vi "main.vi"() -> ()   [LabVIEW 2015, in "example_01.lvlib"]
uses:
  example_01.lvlib
  _controls/recipes.ctl
  _controls/manual_actions.ctl
  lv-recipe-machine/public/_controls/configuration.ctl
  _controls/step_data.ctl
  lv-recipe-machine/public/_controls/mode.ctl
  lv-recipe-machine/lv-recipe-machine.lvlib
panel:
  out "error":errorcluster
  in  "refresh_rate_ms":i32=-1
  out "comparison":bool
  in  "wait_time_ms":i32=1000
  in  "stop":bool
  in  "manual_action":T1=enum."manual_test_random"
  in  "execute":bool
  in  "recipe":T2=enum."simple_random_and_wait"
  in  "resume":bool
  in  "abort":bool
  in  "pause":bool
  in  "start":bool
  in  "manual_mode":bool
  in  "automatic_mode":bool
  out "wait_elapsed_time":dbl format="%<%H:%M:%S%3u>t"
  out "recipe_elapsed_time":dbl format="%<%H:%M:%S>t"
  out "random_data":dbl
  out "action_step":string
  out "state":string
  out "mode":string
  in  "events":i32(listbox)=-1
  # "Manual Inputs"
  # "Automatic Inputs"
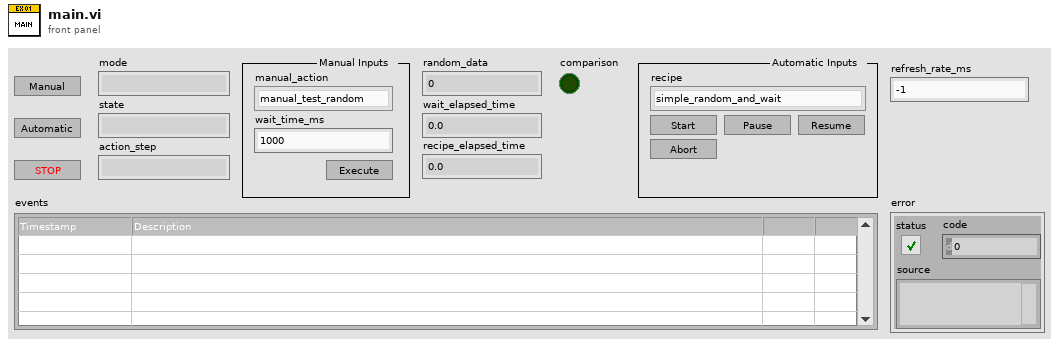
[diagram p1: front panel]
types:
  T1 = typedef "example_01.lvlib/manual_actions.ctl" = enum16{"<manual_action>", "manual_test_random", "manual_test_comparison", "manual_test_wait", "<null>"}
  T2 = typedef "example_01.lvlib/recipes.ctl" = enum16{"<recipes>", "simple_random_and_wait", "simple_random_and_test", "intermediate_fixed_continuous", "intermediate_test_with_continuous_fail", "<null>"}
  T3 = typedef "lv-recipe-machine.lvlib/configuration.ctl" = cluster{"max_processes":i32}
  T4 = typedef "lv-recipe-machine.lvlib/references.ctl" = cluster{"semaphore":T5, "input_queue":refnum<queue>, "output_queue":refnum<queue>, "data_dvr":refnum<data-value>, "stop_notifier":refnum<notifier>, "waitgroup_dvr":refnum<data-value>, "change_in_event":refnum<user-event>, "change_out_event":refnum<user-event>, "status_event":refnum<user-event>}
  T5 = typedef "Semaphore RefNum" = refnum<k1>
  T6 = typedef "example_01.lvlib/step_data.ctl" = cluster{"data":variant, "step":string}
  T7 = typedef "lv-recipe-machine.lvlib/mode.ctl" = enum16{"<mode>", "manual", "automatic", "<null>"}
  T8 = typedef "lv-recipe-machine.lvlib/status.ctl" = cluster{"mode":T7, "manual_state":T9, "automatic_state":T10, "step":string, "auto_elapsed_time":dbl}
  T9 = typedef "lv-recipe-machine.lvlib/manual_state.ctl" = enum16{"<manual_state>", "failed", "action", "running", "idle", "<null>"}
  T10 = typedef "lv-recipe-machine.lvlib/automatic_state.ctl" = enum16{"<automatic_state>", "failed", "idle", "running", "paused", "transition", "stopped", "<null>"}
  T11 = typedef "lv-recipe-machine.lvlib/recipe_step.ctl" = cluster{"step":string, "data":variant}
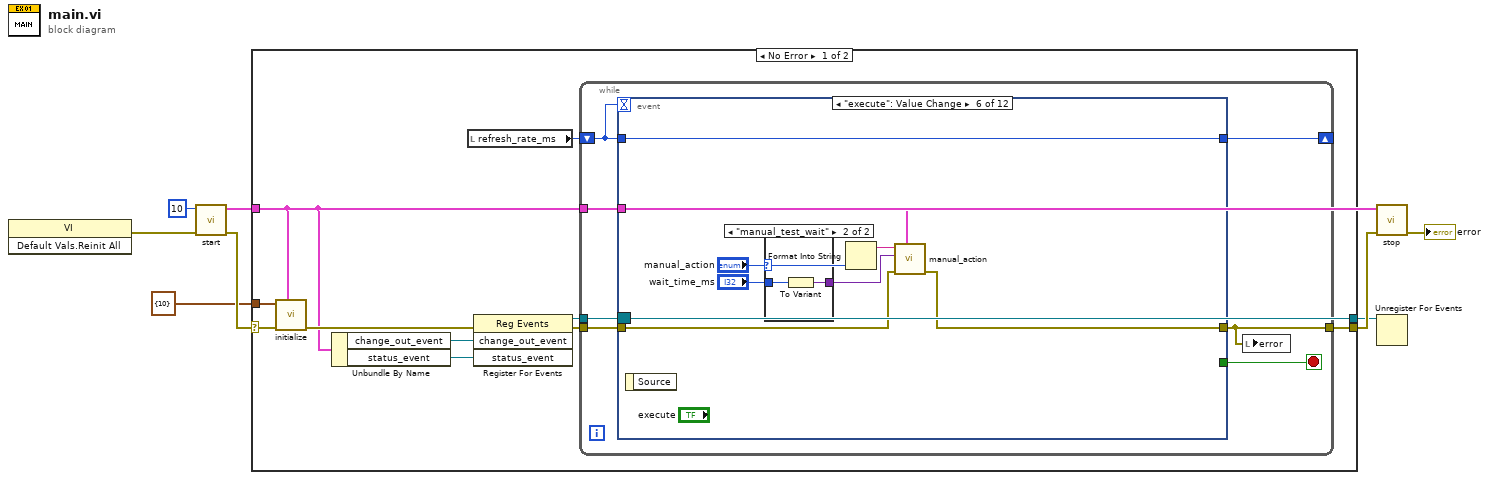
[diagram p0: block diagram]
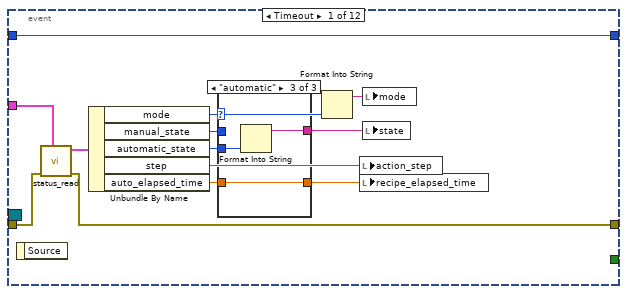
[diagram p2: hidden frame]
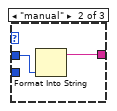
[diagram p4: hidden frame]
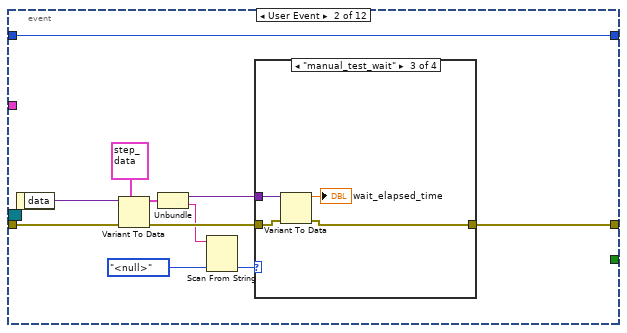
[diagram p5: hidden frame]
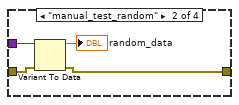
[diagram p7: hidden frame]
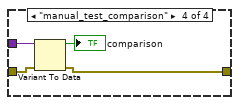
[diagram p8: hidden frame]
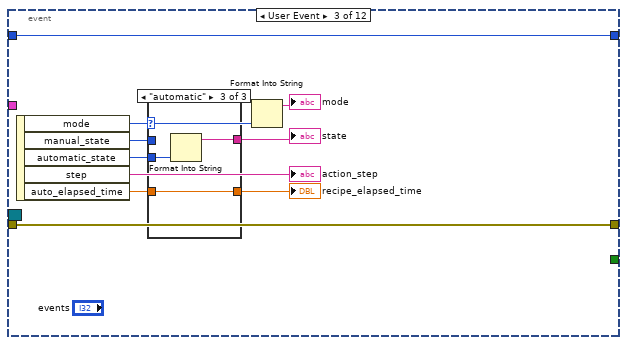
[diagram p9: hidden frame]
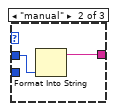
[diagram p11: hidden frame]
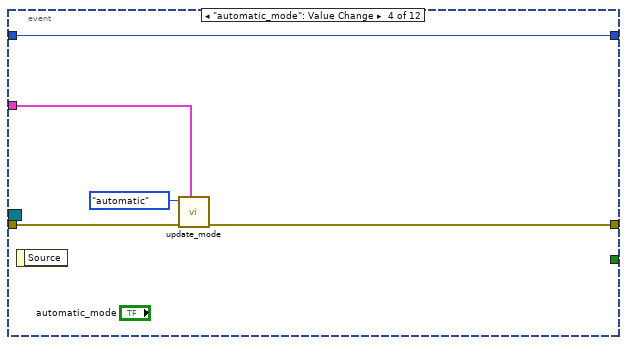
[diagram p12: hidden frame]
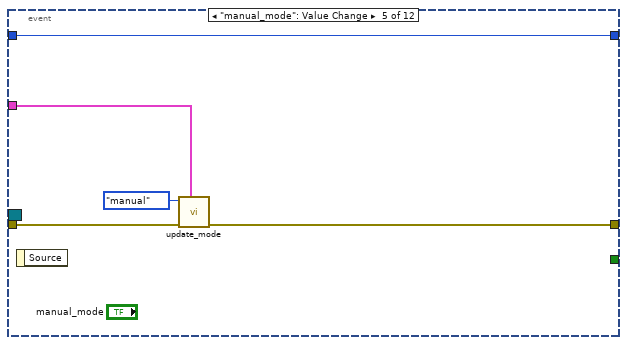
[diagram p13: hidden frame]
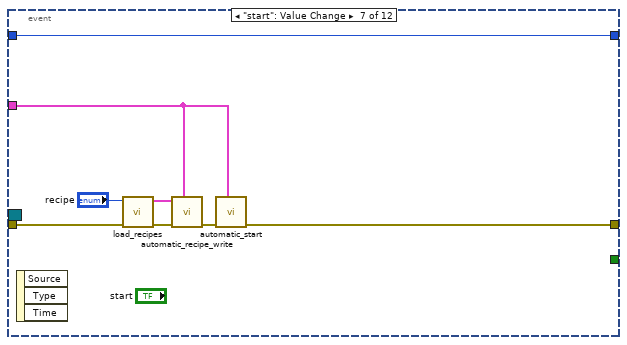
[diagram p15: hidden frame]
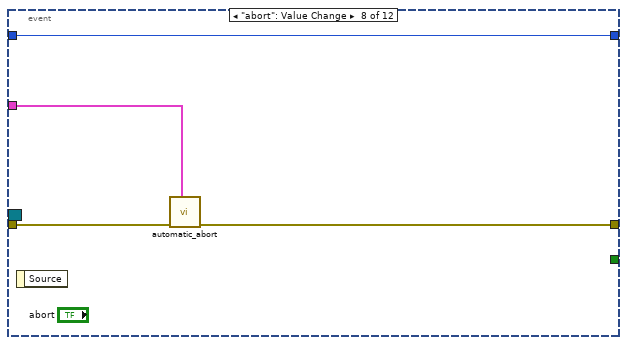
[diagram p16: hidden frame]
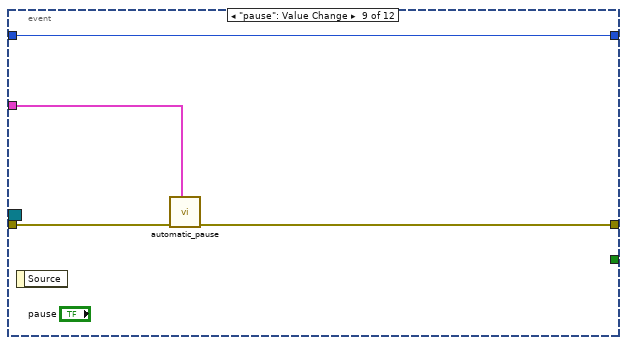
[diagram p17: hidden frame]
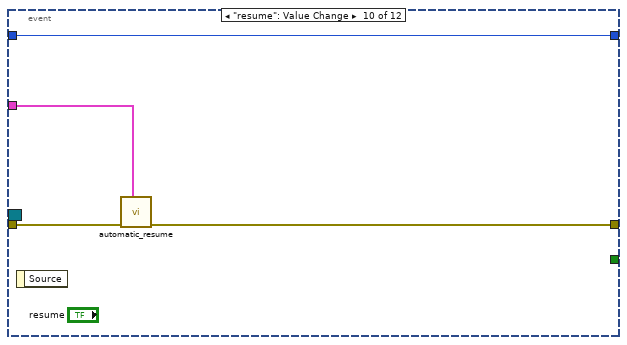
[diagram p18: hidden frame]
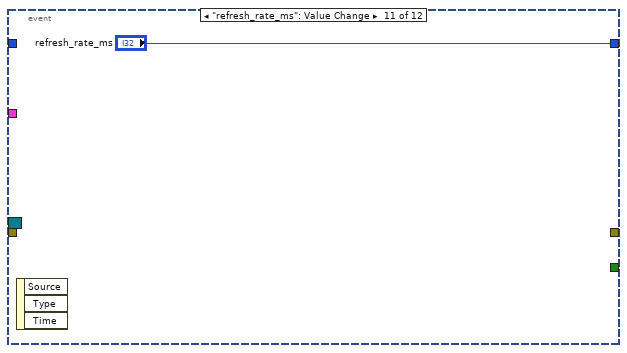
[diagram p19: hidden frame]
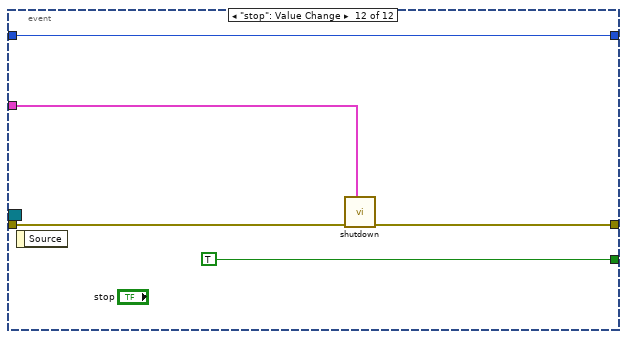
[diagram p20: hidden frame]
diagram:
  n1 = invoke class="VI" method="Default Vals.Reinit All"() -> (error out=w7:errorcluster)  [unwired: 3 in, 2 out]
  n2 = call "start.vi"("error in (no error)"=w7, "queue_size"=10) -> ("error out"=w4:errorcluster, "references"=w6:T4)  [unwired: 8 in]
  n3 = case shown="No Error" w4 {
    selector: w4 -> [w12 w129]
    tunnel: [w17 w129] -> w8
    tunnel: w6 -> [w10 _]
    tunnel: [w14 _] -> w5
    tunnel: T3 {"max_processes"=10} ("configuration") -> [w11 _]
    frame No Error {
      n4 = call "initialize.vi"("references"=w10, "error in (no error)"=w12, "configuration"=w11) -> ("error out"=w18:errorcluster)  [unwired: 8 in]
      n5 = Unbundle By Name(w10) -> ("change_out_event"=w15:refnum<user-event>, "status_event"=w13:refnum<user-event>)
      n6 = local read "refresh_rate_ms"() -> (w9:i32)
      n7 = register-events(error in=w18, w15, w13) -> (reference out=w14:refnum<event-registration>, error out=w16:errorcluster)  [unwired: 1 in]
      n8 = while {
        tunnel: w16 -> [w25]
        tunnel: [w21] -> w17
        tunnel: w10 -> [w23]
        tunnel: w14 -> [w22]
        shift-right: [w20] -> _
        shift-left: w9 -> [w19]
        stop <- w24 stop-if-true
        n9 = event shown="[5] \"execute\": Value Change" {
          selector: w22 -> [_ _ _ _ _ _ _ _ _ _ _ _]
          dyn-events: _ -> [_ _ _ _ _ _ _ _ _ _ _ _]
          timeout: w19 -> [_ _ _ _ _ _ _ _ _ _ _ _]
          tunnel: w25 -> [w38 w53 w77 w86 w91 w100 w109 w114 w118 w122 _ w126]
          tunnel: [w37 w52 w77 w87 w92 w98 w104 w112 w116 w120 _ w125] -> w21
          tunnel: [_ _ _ _ _ _ _ _ _ _ _ TRUE] -> w24
          tunnel: w23 -> [w36 _ _ w85 w90 w97 w105 w113 w117 w121 _ w124]
          tunnel: w19 -> [w28 w51 w71 w83 w88 w93 w103 w111 w115 w119 _ w127]
          tunnel: [w28 w51 w71 w83 w88 w93 w103 w111 w115 w119 "refresh_rate_ms" w127] -> w20
          event Timeout {
            n10 = event-data() -> ()  [unwired: 1 in, 1 out]
            n11 = call "status_read.vi"("references"=w36, "error in (no error)"=w38) -> ("error out"=w37:errorcluster, "status"=w35:T8)  [unwired: 8 in]
            n12 = Unbundle By Name(w35) -> ("mode"=w32:T7, "manual_state"=w34:T9, "automatic_state"=w33:T10, "step"=w29:string, "auto_elapsed_time"=w27:dbl)
            n13 = case shown="\"automatic\"" w32 {
              tunnel: w34 -> [_ w40 _]
              tunnel: w33 -> [_ _ w42]
              tunnel: [_ w39 w43] -> w30
              tunnel: w27 -> [_ _ w41]
              tunnel: [_ _ w41] -> w26
              frame Default {
              }
              frame "manual" {
                n14 = Format Into String(w40) -> (resulting string=w39:string)  [unwired: 3 in, 1 out]
              }
              frame "automatic" {
                n15 = Format Into String(w42) -> (resulting string=w43:string)  [unwired: 3 in, 1 out]
              }
            }
            n16 = Format Into String(w32) -> (resulting string=w31:string)  [unwired: 3 in, 1 out]
            n17 = local write "action_step"(w29) -> ()
            n18 = local write "recipe_elapsed_time"(w26) -> ()
            n19 = local write "mode"(w31) -> ()
            n20 = local write "state"(w30) -> ()
          }
          event User Event {
            n21 = event-data() -> ("data"=w54:variant)  [unwired: 1 in]
            n22 = Variant To Data(error in=w53, type=T6 {"data"=variant, "step"=""}, Variant=w54) -> (data=w49:T6, error out=w48:errorcluster)
            n23 = Unbundle(w49) -> ("data"=w45:variant, "step"=w44:string)
            n24 = Scan From String(input string=w44, default 1=manual_actions."<null>" ("manual_action")) -> (output 1=w46:T1)  [unwired: 3 in, 3 out]
            n25 = case shown="\"manual_test_wait\"" w46 {
              tunnel: w48 -> [w55 w59 w63 w67]
              tunnel: w45 -> [_ w58 w62 w66]
              tunnel: [w55 w56 w61 w65] -> w52
              frame Default {
              }
              frame "manual_test_random" {
                n26 = Variant To Data(error in=w59, Variant=w58) -> (data=→"random_data":dbl, error out=w56:errorcluster)  [unwired: 1 in]
              }
              frame "manual_test_wait" {
                n27 = Variant To Data(error in=w63, Variant=w62) -> (data=→"wait_elapsed_time":dbl, error out=w61:errorcluster)  [unwired: 1 in]
              }
              frame "manual_test_comparison" {
                n28 = Variant To Data(error in=w67, Variant=w66) -> (data=→"comparison":bool, error out=w65:errorcluster)  [unwired: 1 in]
              }
            }
          }
          event User Event {
            n29 = event-data() -> ("mode"=w73:T7, "manual_state"=w76:T9, "automatic_state"=w75:T10, "step"=→"action_step":string, "auto_elapsed_time"=w69:dbl)  [unwired: 1 in]
            n30 = case shown="\"automatic\"" w73 {
              tunnel: w76 -> [_ w78 _]
              tunnel: w75 -> [_ _ w81]
              tunnel: [_ w79 w82] -> w74
              tunnel: w69 -> [_ _ w80]
              tunnel: [_ _ w80] -> w68
              frame Default {
              }
              frame "manual" {
                n31 = Format Into String(w78) -> (resulting string=w79:string)  [unwired: 3 in, 1 out]
              }
              frame "automatic" {
                n32 = Format Into String(w81) -> (resulting string=w82:string)  [unwired: 3 in, 1 out]
              }
            }
            "state" <- w74
            "recipe_elapsed_time" <- w68
            n33 = Format Into String(w73) -> (resulting string=→"mode":string)  [unwired: 3 in, 1 out]
          }
          event "automatic_mode": Value Change {
            n34 = event-data() -> ()  [unwired: 1 in, 1 out]
            n35 = call "update_mode.vi"("references"=w85, "error in (no error)"=w86, "mode"=mode."automatic") -> ("error out"=w87:errorcluster)  [unwired: 8 in]
          }
          event "manual_mode": Value Change {
            n36 = event-data() -> ()  [unwired: 1 in, 1 out]
            n37 = call "update_mode.vi"("references"=w90, "error in (no error)"=w91, "mode"=mode."manual") -> ("error out"=w92:errorcluster)  [unwired: 8 in]
          }
          event "execute": Value Change {
            n38 = event-data() -> ()  [unwired: 1 in, 1 out]
            n39 = case shown="\"manual_test_wait\"" "manual_action" {
              tunnel: "wait_time_ms" -> [_ w102]
              tunnel: [_ w101] -> w94
              frame Default {
              }
              frame "manual_test_wait" {
                n40 = To Variant(anything=w102) -> (Variant=w101:variant)
              }
            }
            n41 = Format Into String("manual_action") -> (resulting string=w99:string)  [unwired: 3 in, 1 out]
            n42 = call "manual_action.vi"("references"=w97, "error in (no error)"=w100, "data"=w94, "step"=w99) -> ("error out"=w98:errorcluster)  [unwired: 7 in]
          }
          event "start": Value Change {
            n43 = event-data() -> ()  [unwired: 1 in, 3 out]
            n44 = call "load_recipes.vi"("error in (no error)"=w109, "recipe"="recipe") -> ("error out"=w107:errorcluster, "recipe []"=w108:T11[])  [unwired: 8 in]
            n45 = call "automatic_recipe_write.vi"("references"=w105, "error in (no error)"=w107, "recipe []"=w108) -> ("error out"=w106:errorcluster)  [unwired: 8 in]
            n46 = call "automatic_start.vi"("references"=w105, "error in (no error)"=w106) -> ("error out"=w104:errorcluster)  [unwired: 9 in]
          }
          event "abort": Value Change {
            n47 = event-data() -> ()  [unwired: 1 in, 1 out]
            n48 = call "automatic_abort.vi"("references"=w113, "error in (no error)"=w114) -> ("error out"=w112:errorcluster)  [unwired: 9 in]
          }
          event "pause": Value Change {
            n49 = event-data() -> ()  [unwired: 1 in, 1 out]
            n50 = call "automatic_pause.vi"("references"=w117, "error in (no error)"=w118) -> ("error out"=w116:errorcluster)  [unwired: 9 in]
          }
          event "resume": Value Change {
            n51 = event-data() -> ()  [unwired: 1 in, 1 out]
            n52 = call "automatic_resume.vi"("references"=w121, "error in (no error)"=w122) -> ("error out"=w120:errorcluster)  [unwired: 9 in]
          }
          event "refresh_rate_ms": Value Change {
            n53 = event-data() -> ()  [unwired: 1 in, 3 out]
          }
          event "stop": Value Change {
            n54 = event-data() -> ()  [unwired: 1 in, 1 out]
            n55 = call "shutdown.vi"("references"=w124, "error in (no error)"=w126) -> ("error out"=w125:errorcluster)  [unwired: 8 in, 1 out]
          }
        }
        n56 = local write "error"(w21) -> ()
      }
    }
    frame Error {
    }
  }
  n57 = call "stop.vi"("error in (no error)"=w8, "references"=w6) -> ("error out"=→"error":errorcluster)  [unwired: 9 in]
  n58 = Unregister For Events(event registration refnum=w5) -> ()  [unwired: 1 in, 1 out]
